vi "OutputMesssageExample.vi"(5 "Sequence Context":refnum<k7>) -> (0 "error out":errorcluster)   [LabVIEW 2013]
panel:
  out "While Loop Index":i32
  # "This VI Generates an output Message everytime the while loop index is a multiple of 10."
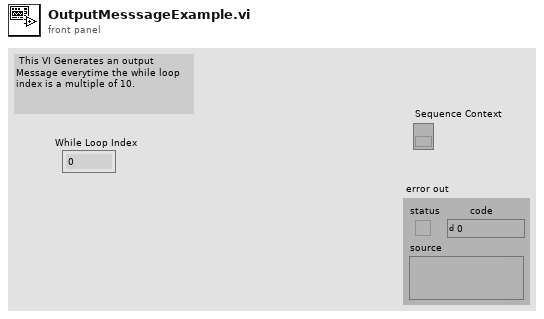
[diagram p1: front panel]
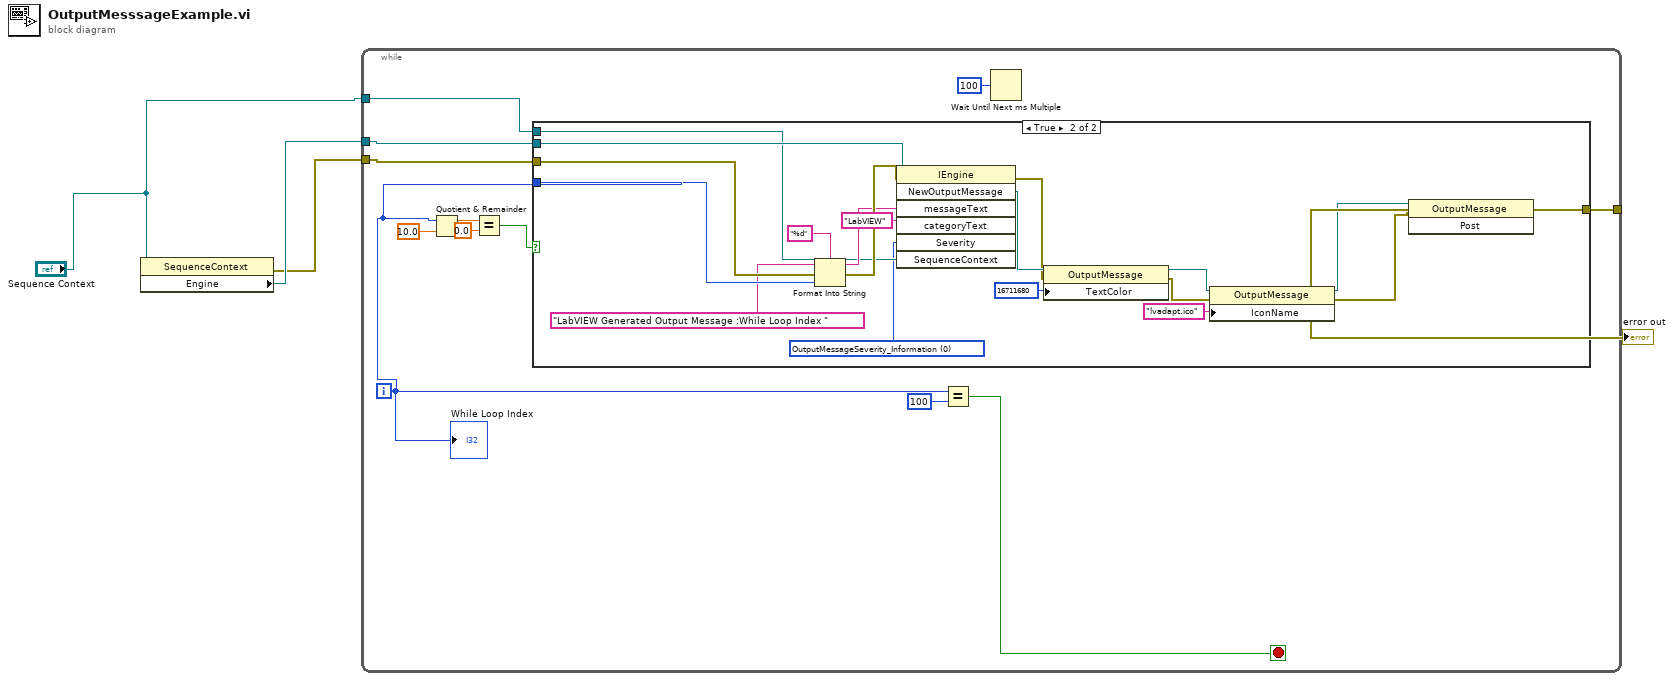
[diagram p0: block diagram]
diagram:
  n1 = property class="SequenceContext"(reference="Sequence Context") -> (error out=w3:errorcluster, "Engine"=w4:refnum<k7>)  [unwired: 1 in, 1 out]
  n2 = while {
    tunnel: w4 -> [w9]
    tunnel: w3 -> [w8]
    tunnel: "Sequence Context" -> [w7]
    tunnel: [w5] -> w1
    i -> [w6]
    stop <- w14 stop-if-true
    n3 = Quotient & Remainder(x=w6, y=10.0) -> (x-y*floor(x/y)=w12:dbl)  [unwired: 1 out]
    n4 = Equal?(x=w12, y=0.0) -> (x = y?=w10:bool)
    n5 = case shown="True" w10 {
      tunnel: w6 -> [_ w33]
      tunnel: w9 -> [_ w36]
      tunnel: w8 -> [w17 w34]
      tunnel: w7 -> [_ w28]
      tunnel: [w17 w26] -> w5
      frame False {
      }
      frame True {
        w27 = 0 items=["OutputMessageSeverity_Information", "OutputMessageSeverity_Warning", "OutputMessageSeverity_Error"] ("Severity")
        n6 = Format Into String(format string="%d", initial string="LabVIEW Generated Output Message :While Loop Index ", error in=w34, w33) -> (resulting string=w30:string, error out=w31:errorcluster)
        n7 = invoke class="IEngine" method="NewOutputMessage"(reference=w36, error in=w31, "messageText"=w30, "categoryText"="LabVIEW", "Severity"=w27, "SequenceContext"=w28) -> (error out=w24:errorcluster, "NewOutputMessage"=w25:refnum<k7>)  [unwired: 1 in, 5 out]
        n8 = property class="OutputMessage"(reference=w25, error in=w24, "TextColor"=16711680) -> (reference out=w21:refnum<k7>, error out=w22:errorcluster)
        n9 = property class="OutputMessage"(reference=w21, error in=w22, "IconName"="lvadapt.ico") -> (reference out=w20:refnum<k7>, error out=w19:errorcluster)
        n10 = invoke class="OutputMessage" method="Post"(reference=w20, error in=w19) -> (error out=w26:errorcluster)  [unwired: 1 in, 2 out]
      }
    }
    n11 = Equal?(x=w6, y=100) -> (x = y?=w14:bool)
    n12 = Wait Until Next ms Multiple(millisecond multiple=u32 100) -> ()  [unwired: 1 out]
    "While Loop Index" <- w6
  }
  "error out" <- w1
